vi "Initialize.vi"(8 "error in (no error)":errorcluster, 11 "initialization in":refnum<class "statemachine.lvclass">) -> (0 "error out":errorcluster, 3 "initialization out":refnum<class "statemachine.lvclass">)   [LabVIEW 2020, in "eos.lvlib" / "statemachine.lvclass"]
uses:
  statemachine.lvclass
  statemachine.lvclass/statemachine.ctl
  interfaces/initialization/initializable.lvclass
  C:/Projects/LVOS/EngineeringOS/source/interfaces/state/state.lvclass
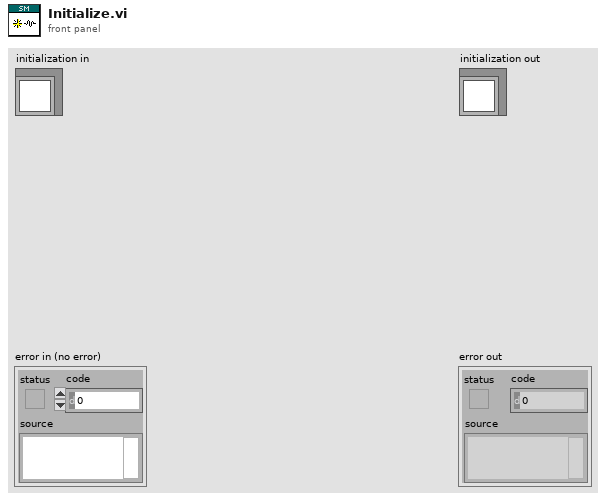
[diagram p1: front panel]
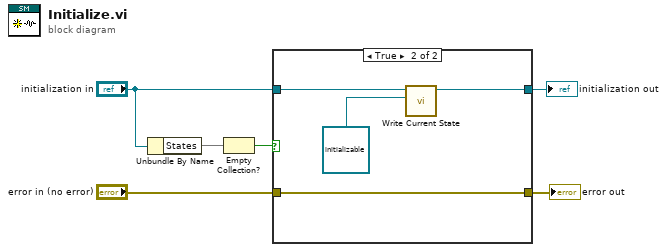
[diagram p0: block diagram]
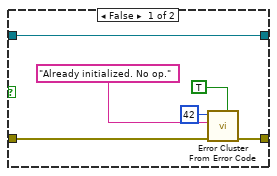
[diagram p2: hidden frame]
diagram:
  n1 = Unbundle By Name("initialization in") -> ("States"=w6:set{refnum<class "state.lvclass">})
  n2 = Empty Collection?(1:w6) -> (0:w5:bool)
  n3 = case shown="True" w5 {
    tunnel: [w12 w16] -> w3
    tunnel: "error in (no error)" -> [w11 w16]
    tunnel: "initialization in" -> [w7 w13]
    tunnel: [w7 w14] -> w1
    frame False {
      n4 = call <vilib>:"Error Cluster From Error Code.vi"("is warning? (False)"=TRUE, "error in (no error)"=w11, "error message (\"\")"="Already initialized. No op." ("error message (\"\")"), "error code (0)"=42) -> ("error out"=w12:errorcluster)  [unwired: 5 in]
    }
    frame True {
      n5 = call "Write Current State.vi"("Current State"=refnum<class "initializable.lvclass"> refnum ("eos.lvlib:initializable.lvclass"), "statemachine in"=w13) -> ("statemachine out"=w14:refnum<class "statemachine.lvclass">)  [unwired: 9 in]
    }
  }
  "error out" <- w3
  "initialization out" <- w1
